vi "Total External Actuator Data.vi"(0 "error in":errorcluster) -> (1 "Left Data":dbl[](array[numeric]), 2 "Right Data":dbl[](array[numeric]), 3 "error out":errorcluster)   [LabVIEW 2009]
uses:
  Actuator Measurment Actions.ctl
  Data Access Objects/External Actuators/External Actuator Id.ctl
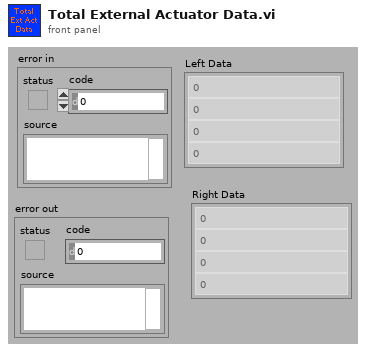
[diagram p1: front panel]
types:
  T1 = typedef "External Actuator Id.ctl" = enum16{"Left", "Right"}
  T2 = typedef "Actuator Measurment Actions.ctl" = enum16{"Set  Data", "Get", "Init"}
  T3 = typedef "External Actuator Data Type.ctl" = cluster{"Command":dbl, "LVDT":dbl, "Load Cell":dbl, "Command\nReturn":dbl}
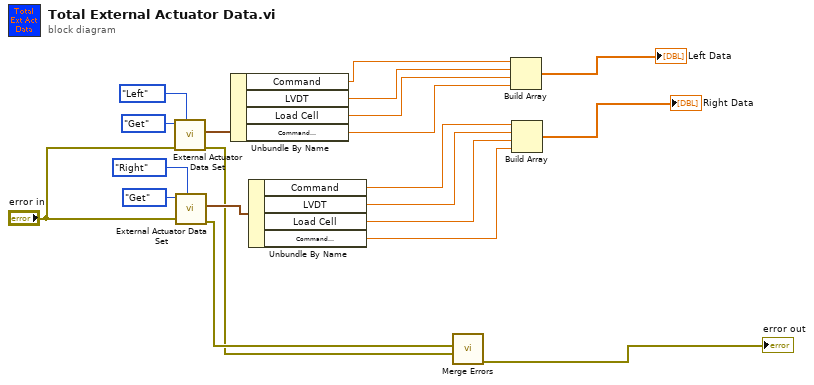
[diagram p0: block diagram]
diagram:
  n1 = call "External Actuator Data Set.vi"("Selected Actuator"=External_Actuator_Id."Left", "error in (no error)"="error in", "Measurement Actions"=Actuator_Measurment_Actions."Get") -> ("error out"=w1:errorcluster, "Actuator Data Out"=w8:T3)  [unwired: 6 in, 1 out]
  n2 = call "External Actuator Data Set.vi"("Selected Actuator"=External_Actuator_Id."Right", "error in (no error)"="error in", "Measurement Actions"=Actuator_Measurment_Actions."Get") -> ("error out"=w10:errorcluster, "Actuator Data Out"=w9:T3)  [unwired: 6 in, 1 out]
  n3 = Unbundle By Name(w8) -> ("Command"=w11:dbl, "LVDT"=w12:dbl, "Load Cell"=w13:dbl, "Command\nReturn"=w19:dbl)
  n4 = Unbundle By Name(w9) -> ("Command"=w14:dbl, "LVDT"=w15:dbl, "Load Cell"=w16:dbl, "Command\nReturn"=w20:dbl)
  n5 = call <vilib>:"Merge Errors.vi"("error in 3 (no error)"=w1, "error in 2 (no error)"=w10) -> ("error out"=→"error out":errorcluster)  [unwired: 5 in]
  n6 = Build Array(w11, w12, w13, w19) -> (→"Left Data":dbl[])
  n7 = Build Array(w14, w15, w16, w20) -> (→"Right Data":dbl[])
